vi "Send Trace Query Options.vi"(6 "Options":T1={"interpolate data (F)"=FALSE, "extrapolate to now (F)"=FALSE, "remove data breaks (F)"=FALSE, "interpolation interval (1 s)"=1.0, "maintain trending info (T)"=TRUE} {"interpolation interval (1 s)" min=0.0 format="%0.2f"}, 7 "Message Priority (Normal)":T3=enum."Normal", 8 "error in (no error)":errorcluster, 9 "Time Interval":T2 {"Stop Time" format="%<%H:%M:%S\n%Y/%m/%d>T"; "Start Time" format="%<%H:%M:%S\n%Y/%m/%d>T"}, 10 "Max Points per Trace (all)":i32=-1, 11 "Message Enqueuer":refnum<class "Message Enqueuer.lvclass">) -> (0 "error out":errorcluster, 3 "Message Enqueuer out":refnum<class "Message Enqueuer.lvclass">)   [LabVIEW 2015, in "BNT_DSCXtGraph.lvlib" / "Trace Query Options Msg.lvclass"]
doc: "This VI sends the message to an actor."
uses:
  Trace Query Options Msg.lvclass
  <vilib>/ActorFramework/Message Enqueuer/Message Enqueuer.lvclass
  <vilib>/ActorFramework/Message Enqueuer/Message Priority.ctl
  Trace Query Options Msg.lvclass/Trace Query Options Msg.ctl
  <vilib>/ActorFramework/Message Enqueuer/Message Enqueuer.lvclass/Message Enqueuer.ctl
  <vilib>/ActorFramework/Message Priority Queue/Priority Enqueue.vi
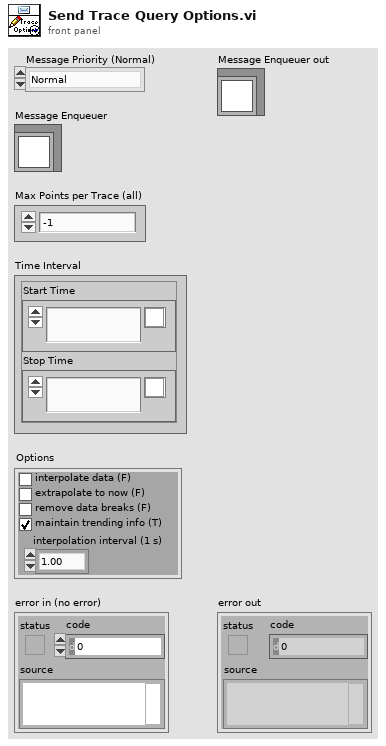
[diagram p1: front panel]
types:
  T1 = cluster{"interpolate data (F)":bool, "extrapolate to now (F)":bool, "remove data breaks (F)":bool, "interpolation interval (1 s)":dbl, "maintain trending info (T)":bool}
  T2 = cluster{"Start Time":timestamp, "Stop Time":timestamp}
  T3 = typedef "Actor Framework.lvlib/Message Enqueuer.lvclass/Message Priority.ctl" = enum16{"Low", "Normal", "High"}
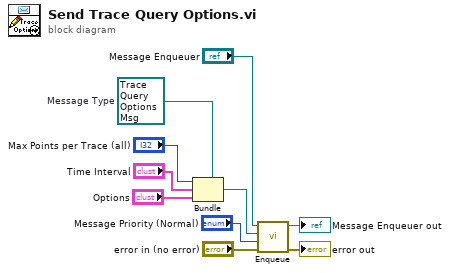
[diagram p0: block diagram]
diagram:
  w7 = refnum<class "Trace Query Options Msg.lvclass"> refnum  # Message Type
  n1 = Bundle(cluster=w7, "Max Points per Trace (all)", "Time Interval", "Options") -> (w6:refnum<class "Trace Query Options Msg.lvclass">)
  n2 = call <vilib>:"Enqueue.vi"("error in (no error)"="error in (no error)", "Message Priority (Normal)"="Message Priority (Normal)", "Message"=w6, "Message Enqueuer in"="Message Enqueuer") -> ("error out"=→"error out":errorcluster, "Message Enqueuer out"=→"Message Enqueuer out":refnum<class "Message Enqueuer.lvclass">)  [unwired: 6 in]
